vi "PCAN_CLOSE.vi"(8 "error in (no error)":errorcluster) -> (0 "error out":errorcluster, 3 "error":T1 items=["CAN_ERR_OK"=0, "CAN_ERR_XMTFULL"=1, "CAN_ERR_OVERRUN"=2, "CAN_ERR_BUSLIGHT"=4, "CAN_ERR_BUSHEAVY"=8, "CAN_ERR_BUSOFF"=16, "CAN_ERR_QRCVEMPTY"=32, "CAN_ERR_QOVERRUN"=64, "CAN_ERR_QXMTFULL"=128, "CAN_ERR_REGTEST"=256, "CAN_ERR_NOVXD"=512, "CAN_ERR_RESOURCE"=8192, "CAN_ERR_ILLPARAMTYPE"=16384, "CAN_ERR_ILLPARAMVAL"=32768])   [LabVIEW 2016]
uses:
  PCAN_ERROR.ctl
  PCAN_USB.DLL
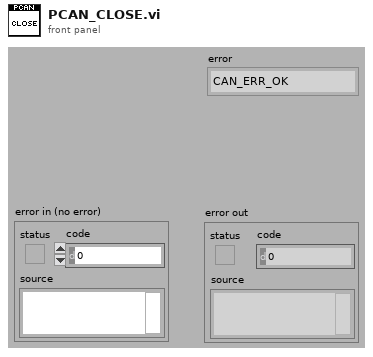
[diagram p1: front panel]
types:
  T1 = typedef "PCAN_ERROR.ctl" = i32
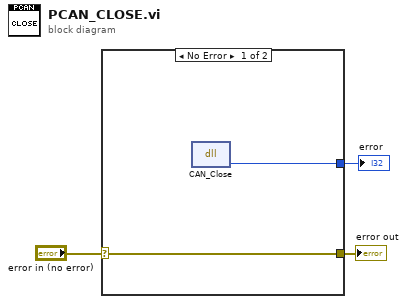
[diagram p0: block diagram]
diagram:
  n1 = case shown="No Error" "error in (no error)" {
    selector: "error in (no error)" -> [w4 w6]
    tunnel: [w5 _] -> w1
    tunnel: [w4 w6] -> w2
    frame No Error {
      n2 = dll-call lib="D:/LabView/08_PCAN&Measurement/PCAN_Driver/PCAN_USB.DLL" fn="CAN_Close"() -> ("return type"=w5:i32)  [unwired: 3 in, 2 out]
    }
    frame Error {
    }
  }
  "error out" <- w2
  "error" <- w1
